vi "QueueDriver.vi"(0 "Queue Name":string, 5 "State":string, 7 "States[]":string[](array[string]), 11 "error in (no error)":errorcluster, 13 "Queue Operations":T1) -> (4 "Dequeued Element":string, 15 "error out":errorcluster)   [LabVIEW 2021, in "Calculator.lvlib"]
doc: "This VI acts as a queue driver , which handles queue operations such as enqueue , dequeue , flush and release."
uses:
  Calculator.lvlib
  Controls/QueueOperations.ctl
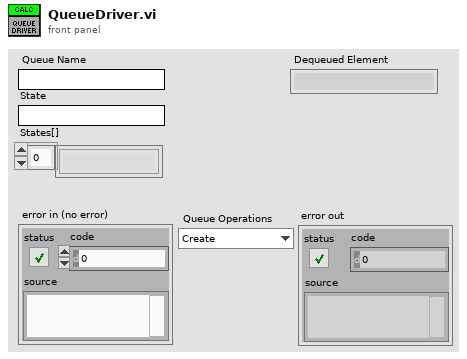
[diagram p1: front panel]
types:
  T1 = typedef "Calculator.lvlib/QueueOperations.ctl" = enum16{"Create", "Enqueue", "EnqueueN", "Enqueue at Top", "Dequeue", "Flush", "Release"}
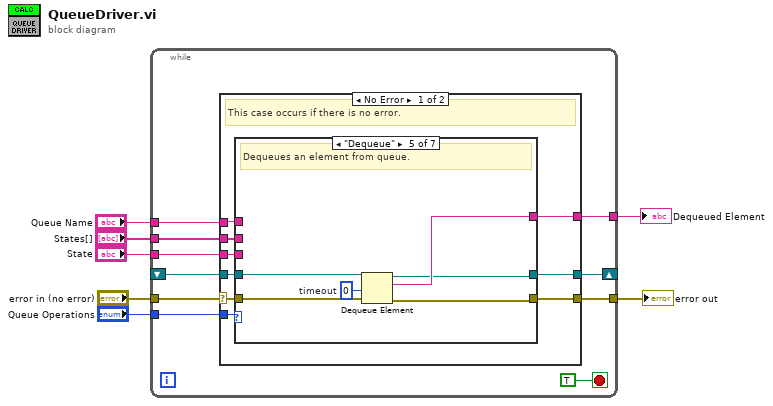
[diagram p0: block diagram]
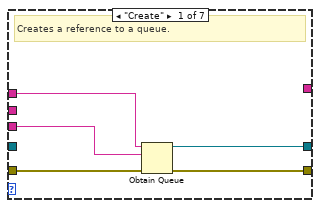
[diagram p2: hidden frame]
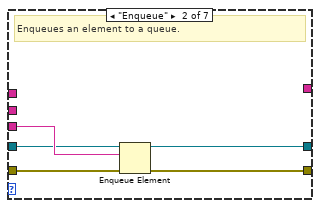
[diagram p3: hidden frame]
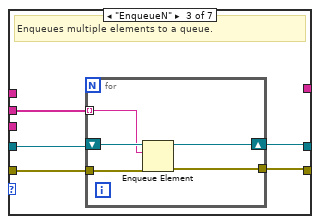
[diagram p4: hidden frame]
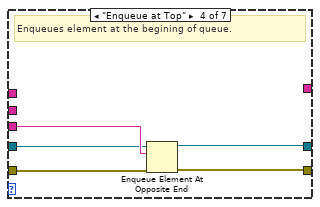
[diagram p5: hidden frame]
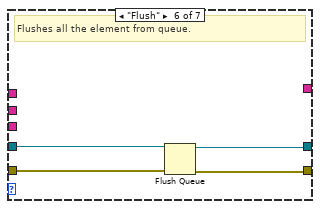
[diagram p6: hidden frame]
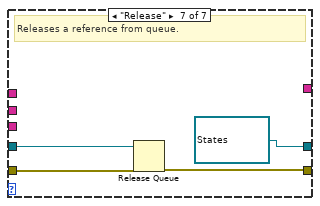
[diagram p7: hidden frame]
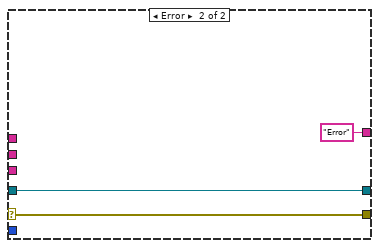
[diagram p8: hidden frame]
diagram:
  n1 = while {
    tunnel: "error in (no error)" -> [w17]
    tunnel: "Queue Operations" -> [w16]
    tunnel: "Queue Name" -> [w15]
    tunnel: [w14] -> w2
    tunnel: "State" -> [w13]
    shift-right: [w12] -> _
    shift-left: _ -> [w11]
    tunnel: [w10] -> w3
    tunnel: "States[]" -> [w8]
    stop <- TRUE stop-if-true
    n2 = case shown="No Error" w17 {
      selector: w17 -> [w24 w67]
      tunnel: w16 -> [w26 _]
      tunnel: w15 -> [w25 _]
      tunnel: [w23 w67] -> w14
      tunnel: w13 -> [w22 _]
      tunnel: [w21 w68] -> w12
      tunnel: w11 -> [w20 w68]
      tunnel: [w19 "Error" ("States")] -> w10
      tunnel: w8 -> [w18 _]
      frame No Error {
        # "This case occurs if there is no error."
        n3 = case shown="\"Dequeue\"" w26 {
          tunnel: w25 -> [w31 _ _ _ _ _ _]
          tunnel: w24 -> [w30 w36 w41 w51 w57 w61 w65]
          tunnel: [w27 w32 w40 w47 w53 w58 w64] -> w23
          tunnel: w22 -> [w29 w35 _ w50 _ _ _]
          tunnel: [w28 w34 w38 w49 w54 w59 refnum<queue> refnum ("queue out")] -> w21
          tunnel: w20 -> [_ w33 w39 w48 w55 w60 w63]
          tunnel: [_ _ _ _ w56 _ _] -> w19
          tunnel: w18 -> [_ _ w37 _ _ _ _]
          frame "Create" {
            # "Creates a reference to a queue."
            n4 = Obtain Queue(name (unnamed)=w31, element data type=w29, error in (no error)=w30) -> (queue out=w28:refnum<queue>, error out=w27:errorcluster)  [unwired: 2 in, 1 out]
          }
          frame "Enqueue" {
            # "Enqueues an element to a queue."
            n5 = Enqueue Element(queue=w33, element=w35, error in (no error)=w36) -> (queue out=w34:refnum<queue>, error out=w32:errorcluster)  [unwired: 1 in, 1 out]
          }
          frame "EnqueueN" {
            # "Enqueues multiple elements to a queue."
            n6 = for {
              tunnel: w41 -> [w46]
              tunnel: [w45] -> w40
              shift-right: [w43] -> w38
              shift-left: w39 -> [w44]
              tunnel: w37 -> [w42] mode=indexing
              n7 = Enqueue Element(queue=w44, element=w42, error in (no error)=w46) -> (queue out=w43:refnum<queue>, error out=w45:errorcluster)  [unwired: 1 in, 1 out]
            }
          }
          frame "Enqueue at Top" {
            # "Enqueues element at the begining of queue."
            n8 = Enqueue Element At Opposite End(queue=w48, element=w50, error in (no error)=w51) -> (queue out=w49:refnum<queue>, error out=w47:errorcluster)  [unwired: 1 in, 1 out]
          }
          frame "Dequeue" {
            w52 = 0  # timeout
            # "Dequeues an element from queue."
            n9 = Dequeue Element(queue=w55, timeout in ms (-1)=w52, error in (no error)=w57) -> (queue out=w54:refnum<queue>, element=w56:string, error out=w53:errorcluster)  [unwired: 1 out]
          }
          frame "Flush" {
            # "Flushes all the element from queue."
            n10 = Flush Queue(queue=w60, error in (no error)=w61) -> (queue out=w59:refnum<queue>, error out=w58:errorcluster)  [unwired: 1 out]
          }
          frame "Release" {
            # "Releases a reference from queue."
            n11 = Release Queue(queue=w63, error in (no error)=w65) -> (error out=w64:errorcluster)  [unwired: 1 in, 2 out]
          }
        }
      }
      frame Error {
      }
    }
  }
  "error out" <- w2
  "Dequeued Element" <- w3
